vi "MotorVI.vi"(6 "stop button":bool, 7 "PWM Channel":u8, 8 "error in (no error)":errorcluster, 9 "Duty Cycle":dbl(slide) scale=-200.0..200.0, 10 "LINX Resource in":T1, 11 "AI1 and AI2 Channels":u8[](array[numeric])) -> (0 "error out":errorcluster, 3 "LINX Resource out":T1)   [LabVIEW 2020]
uses:
  <vilib>/MakerHub/LINX/Private/Type Defs/LINX Ref.ctl
  <vilib>/MakerHub/LINX/Private/Type Defs/Platform.ctl
  <vilib>/MakerHub/LINX/Private/Type Defs/Interface.ctl
  <vilib>/MakerHub/LINX/Private/Device/Type Defs/LINX Device Config.ctl
  <vilib>/MakerHub/LINX/Private/Device/Type Defs/TCP Config.ctl
  <vilib>/MakerHub/LINX/Private/Device/Type Defs/Channels.ctl
  <vilib>/MakerHub/LINX/Public/Peripherals/Digital/Digital Write N Chans.vi
  <vilib>/MakerHub/LINX/Public/Peripherals/PWM/PWM Set Duty Cycle 1 Chan.vi
  <vilib>/MakerHub/LINX/Private/Local IO/LinxDigitalWrite.vi
  <vilib>/MakerHub/LINX/Public/Utilities/Check Channel.vi
  <vilib>/MakerHub/LINX/Private/Utilties/Generate Error.vi
  <vilib>/MakerHub/LINX/Public/Peripherals/PWM/PWM Set Duty Cycle N Chans.vi
  <vilib>/MakerHub/LINX/LMH-LINX.lvlib
  <vilib>/MakerHub/LINX/Private/Device/Device.lvlib
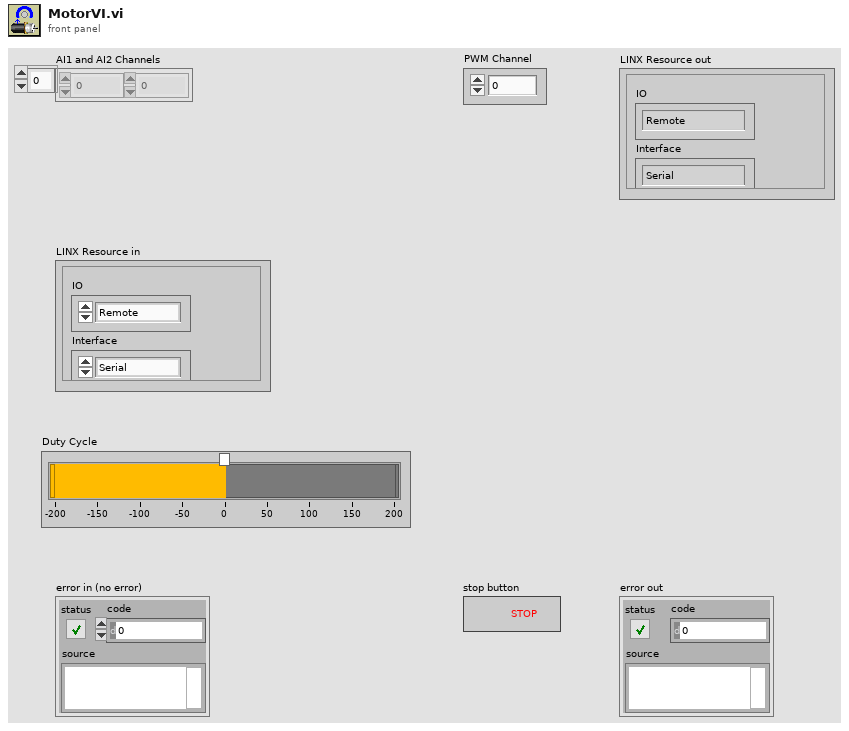
[diagram p1: front panel]
types:
  T1 = typedef "LMH-LINX.lvlib/LINX Ref.ctl" = cluster{"IO":T2, "Interface":T3, "LINX Device Config":T4}
  T2 = typedef "LMH-LINX.lvlib/Platform.ctl" = enum16{"Remote", "Local"}
  T3 = typedef "LMH-LINX.lvlib/Interface.ctl" = enum16{"Serial", "TCP"}
  T4 = typedef "LMH-LINX.lvlib/Device.lvlib/LINX Device Config.ctl" = cluster{"Interface":T3, "COM Port":refnum<visa-resource-name>, "TCP Configuration":T5, "Device Family":u8, "Device ID":u8, "Device Name":string, "TCP Ref":refnum<k5>, "Channels":T6}
  T5 = typedef "LMH-LINX.lvlib/Device.lvlib/TCP Config.ctl" = cluster{"IP Address":string, "Port":u16}
  T6 = typedef "LMH-LINX.lvlib/Channels.ctl" = cluster{"DI":u8[], "DO":u8[], "AI":u8[], "AO":u8[], "PWM":u8[], "QE":u8[], "UART":u8[], "I2C 2":u8[], "SPI":u8[], "CAN":u8[], "Servo":u8[], "AI Ref (V)":dbl, "AI Resolution (Bits)":u8, "AO Ref (V)":dbl, "AO Resolution (Bits)":u8}
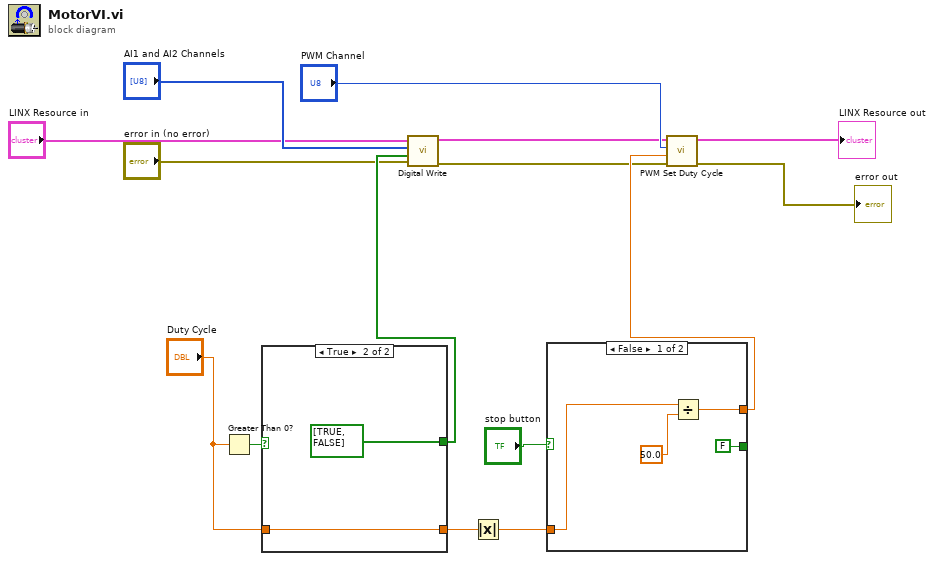
[diagram p0: block diagram]
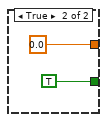
[diagram p2: hidden frame]
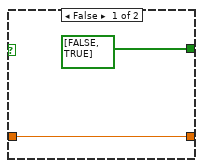
[diagram p3: hidden frame]
diagram:
  n1 = Greater Than 0?(x="Duty Cycle") -> (x > 0?=w7:bool)
  n2 = case shown="True" w7 {
    tunnel: "Duty Cycle" -> [w16 w18]
    tunnel: [bool[] [FALSE, TRUE] bool[] [TRUE, FALSE]] -> w9
    tunnel: [w16 w18] -> w12
    frame False {
    }
    frame True {
    }
  }
  n3 = call-poly <vilib>:"Digital Write.vi"("Error In"="error in (no error)", "Values"=w9, "DO Channels"="AI1 and AI2 Channels", "LINX Resource"="LINX Resource in") -> ("Error Out"=w5:errorcluster, "LINX Resource"=w2:T1)  [unwired: 6 in]
  n4 = Absolute Value(x=w12) -> (abs(x)=w14:dbl)
  n5 = case shown="False" "stop button" {
    tunnel: [FALSE TRUE] -> _
    tunnel: [w22 0.0] -> w13
    tunnel: w14 -> [w20 _]
    frame False {
      n6 = Divide(x=w20, y=50.0) -> (x/y=w22:dbl)
    }
    frame True {
    }
  }
  n7 = call-poly <vilib>:"PWM Set Duty Cycle.vi"("Error In"=w5, "Duty Cycle (0-1)"=w13, "PWM Channel"="PWM Channel", "LINX Resource"=w2) -> ("Error Out"=→"error out":errorcluster, "LINX Resource"=→"LINX Resource out":T1)  [unwired: 6 in]
